vi "读取数据库.vi"(7 "condition":string, 8 "error in (no error)":errorcluster caption="错误输入（无错误）", 9 "database":string="database1.mdb", 10 "显示项":string[](array[string]), 11 "组合框":string(combo)) -> (0 "error out":errorcluster caption="错误输出", 1 "columns":string[](array[string]), 2 "data":variant[][](array[variant]), 3 "表格":string[][](table))   [LabVIEW 2016, in "数据查询.lvlib"]
uses:
  <vilib>/Utility/sysdir.llb/System Directory Type.ctl
  <vilib>/addons/database/Connection.llb/DB Tools Open Connec (String).vi
  <vilib>/addons/database/_DB Variant To Data/Database Variant To Data.xnode
  <vilib>/addons/database/NI_Database_API.lvlib
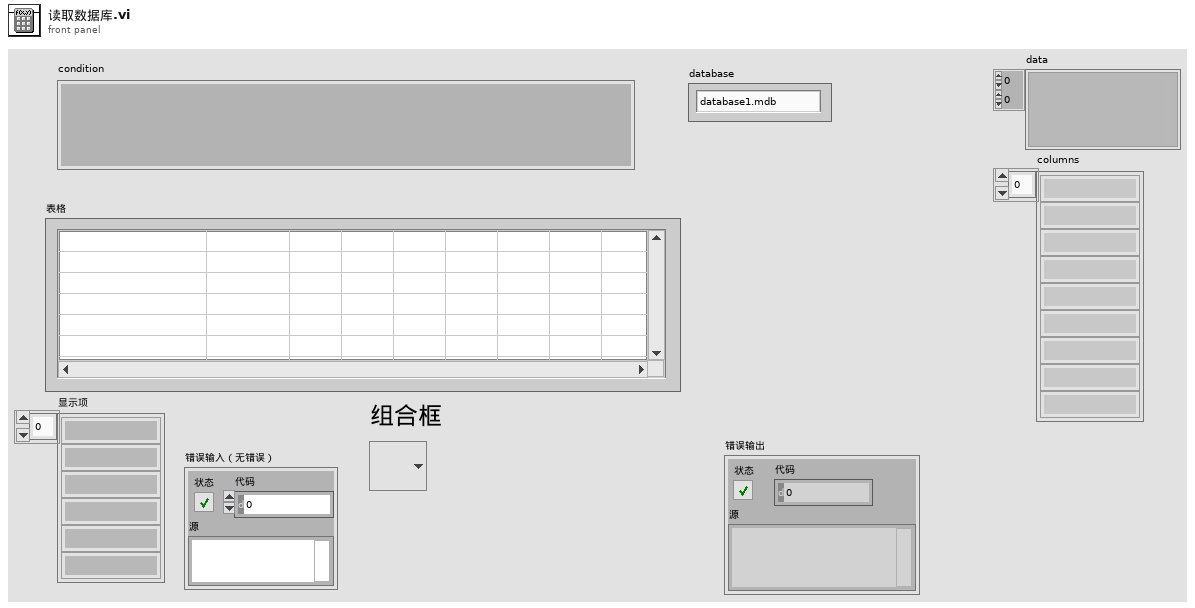
[diagram p1: front panel]
types:
  T1 = typedef "System Directory Type.ctl" = i32
  T2 = typedef "NI_Database_API.lvlib/Conn ObjectReference.ctl" = refnum<k1>
  T3 = typedef "NI_Database_API.lvlib/DB Tools DataTypes.ctl" = enum16{"String", "Long (I32)", "Single (SGL)", "Double (DBL)", "Date/Time", "Binary"}
  T4 = cluster{"name":string, "database data type":T3, "defined size":i32}[]
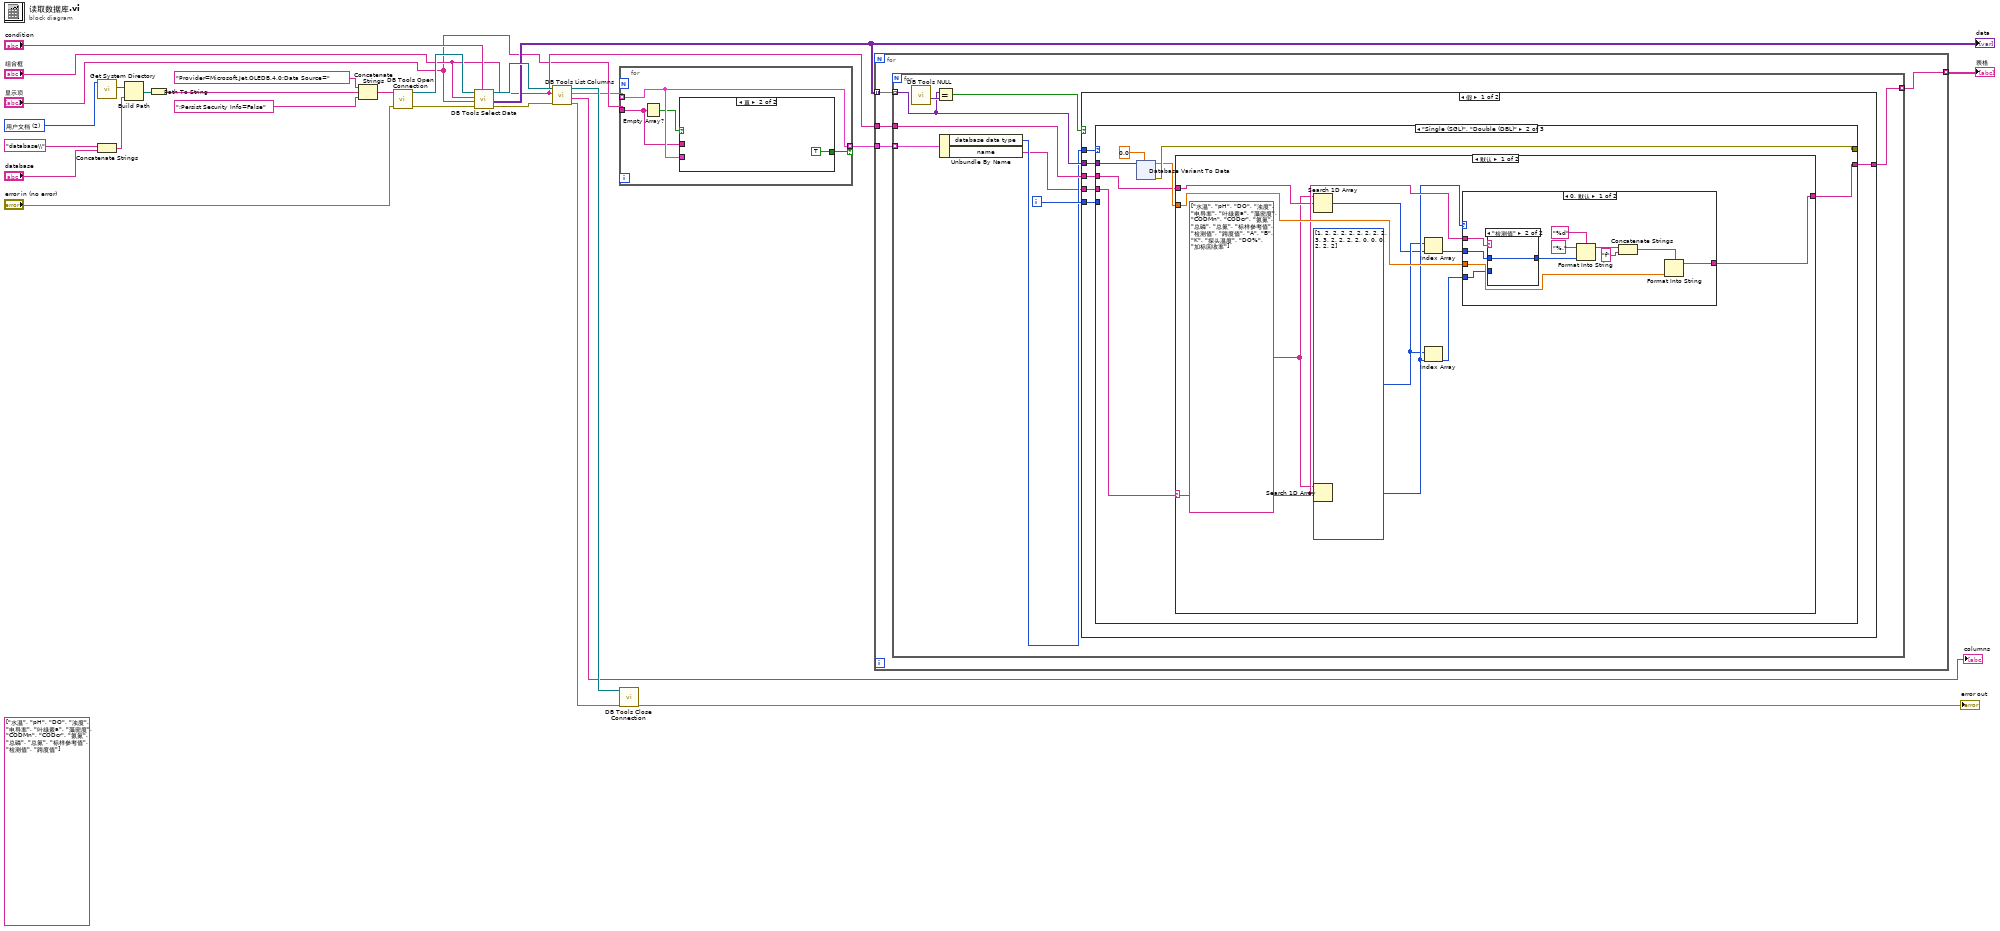
[diagram p0: block diagram]
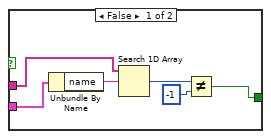
[diagram p2: hidden frame]
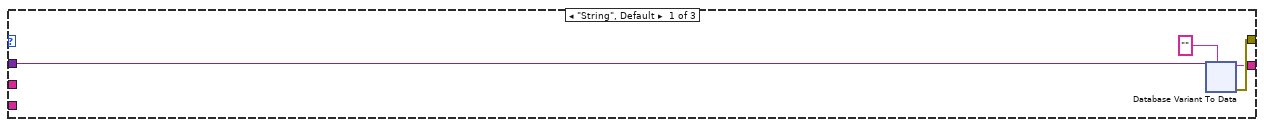
[diagram p3: hidden frame]
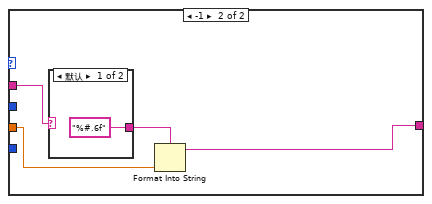
[diagram p5: hidden frame]
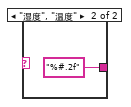
[diagram p6: hidden frame]
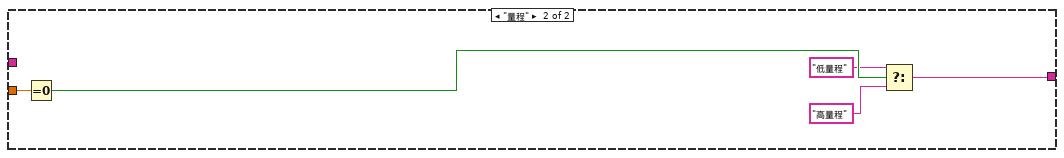
[diagram p7: hidden frame]
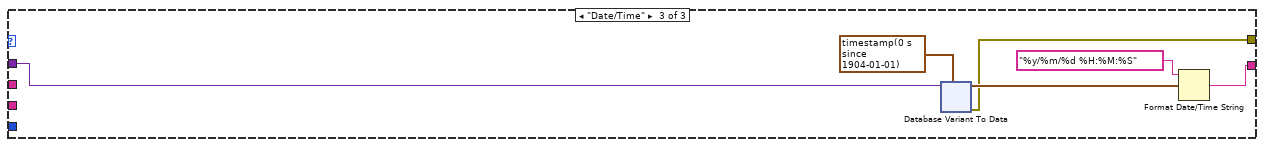
[diagram p8: hidden frame]
diagram:
  (unwired) string[] ["水温", "pH", "DO", "浊度", "电导率", "叶绿素a", "藻密度", "CODMn", "CODcr", "氨氮", "总磷", "总氮", "标样参考值", "检测值", "跨度值"]
  w13 = T1 2 items=["用户目录"=0, "用户桌面"=1, "用户文档"=2, "用户应用程序数据"=3, "用户设置"=4, "用户临时目录"=5, "公共文档"=6, "公共应用程序数据"=7, "公共设置"=8, "公共缓存"=13, "系统核心库"=9, "系统安装库"=10, "应用程序文件"=11, "启动盘根目录"=12] ("system directory type")
  n1 = call <vilib>:"Get System Directory.vi"("system directory type"=w13) -> ("system directory"=w12:path)  [unwired: 10 in]
  n2 = Concatenate Strings("database\\" ("名称或相对路径"), "database") -> (w9:string)
  n3 = Build Path(base path=w12, name or relative path=w9) -> (appended path=w14:path)
  n4 = Path To String(path=w14) -> (string=w15:string)
  n5 = Concatenate Strings("Provider=Microsoft.Jet.OLEDB.4.0;Data Source=", w15, ";Persist Security Info=False") -> (w11:string)
  n6 = call-poly <vilib>:"DB Tools Open Connection.vi"("error in (no error)"="error in (no error)", "connection information"=w11) -> ("error out"=w25:errorcluster, "connection reference"=w26:T2)  [unwired: 6 in]
  n7 = call <vilib>:"DB Tools Select Data.vi"("condition"="condition", "error in (no error)"=w25, "columns"="显示项", "table"="组合框", "connection reference"=w26) -> ("error out"=w24:errorcluster, "data"=w7:variant[][], "connection reference out"=w21:T2)  [unwired: 1 in]
  "data" <- w7
  n8 = call <vilib>:"DB Tools List Columns.vi"("error in (no error)"=w24, "table"="组合框", "connection reference"=w21) -> ("error out"=w18:errorcluster, "columns"=→"columns":string[], "column information"=w2:T4, "connection reference out"=w19:T2)  [unwired: 1 in]
  n9 = for {
    tunnel: w2 -> [w29] mode=indexing
    tunnel: "显示项" -> [w28]
    tunnel: [w29] -> w1 mode=indexing if=w30
    n10 = Empty Array?(array=w28) -> (empty?=w27:bool)
    n11 = case shown="真" w27 {
      tunnel: [w33 TRUE] -> w30
      tunnel: w29 -> [w32 _]
      tunnel: w28 -> [w31 _]
      frame False {
        n12 = Unbundle By Name(w32) -> ("name"=w34:string)
        n13 = Search 1D Array(1D array=w31, element=w34) -> (index of element=w36:i32)  [unwired: 1 in]
        n14 = Not Equal?(x=w36, y=-1) -> (x != y?=w33:bool)
      }
      frame True {
      }
    }
  }
  n15 = call <vilib>:"DB Tools Close Connection.vi"("error in (no error)"=w18, "connection reference"=w19) -> ("error out"=→"error out":errorcluster)  [unwired: 5 in]
  n16 = for {
    tunnel: w7 -> [w41] mode=indexing
    tunnel: w1 -> [w40]
    tunnel: [w39] -> w6 mode=indexing
    tunnel: "组合框" -> [w38]
    n17 = for {
      tunnel: w41 -> [w46] mode=indexing
      tunnel: w40 -> [w50] mode=indexing
      tunnel: [w48] -> w39 mode=indexing
      tunnel: w38 -> [w44]
      i -> [w49]
      n18 = call <vilib>:"DB Tools NULL.vi"() -> ("NULL"=w47:variant)  [unwired: 10 in, 1 out]
      n19 = Equal?(x=w46, y=w47) -> (x = y?=w45:bool)
      n20 = Unbundle By Name(w50) -> ("database data type"=w43:T3, "name"=w42:string)
      n21 = case shown="假" w45 {
        tunnel: w43 -> [w56 _]
        tunnel: w49 -> [w55 _]
        tunnel: [w54 _] -> w48
        tunnel: w42 -> [w53 _]
        tunnel: w46 -> [w52 _]
        tunnel: w44 -> [w51 _]
        frame False {
          n22 = case shown="\"Single (SGL)\", \"Double (DBL)\"" w56 {
            tunnel: w52 -> [w60 w97 w171]
            tunnel: [w57 w98 w167] -> w54
            tunnel: w55 -> [_ _ _]
            tunnel: [w58 w99 w166] -> _
            tunnel: w53 -> [_ w96 _]
            tunnel: w51 -> [_ w93 _]
            frame "String", Default {
              n23 = xnode "Database Variant To Data"("database variant"=w60, "type"="") -> ("data"=w57:string, "error out"=w58:errorcluster)  [unwired: 1 in]
            }
            frame "Single (SGL)", "Double (DBL)" {
              n24 = xnode "Database Variant To Data"("database variant"=w97, "type"=0.0) -> ("data"=w94:dbl, "error out"=w99:errorcluster)  [unwired: 1 in]
              n25 = case shown="默认" w96 {
                selector: w96 -> [w107 _]
                tunnel: w94 -> [w109 w133]
                tunnel: [w108 w129] -> w98
                tunnel: w93 -> [w105 _]
                frame Default {
                  w100 = string[] ["水温", "pH", "DO", "浊度", "电导率", "叶绿素a", "藻密度", "CODMn", "CODcr", "氨氮", "总磷", "总氮", "标样参考值", "检测值", "跨度值", "A", "B", "K", "探头温度", "DO%", "加标回收率"]
                  w104 = i32[] [1, 2, 2, 2, 2, 2, 2, 2, 2, 3, 3, 2, 2, 2, 2, 0, 0, 0, 2, 2, 2]
                  n26 = Search 1D Array(1D array=w100, element=w105) -> (index of element=w103:i32)  [unwired: 1 in]
                  n27 = Search 1D Array(1D array=w100, element=w107) -> (index of element=w106:i32)  [unwired: 1 in]
                  n28 = Index Array(array=w104, index=w103) -> (element=w102:i32)
                  n29 = Index Array(array=w104, index=w106) -> (element=w101:i32)
                  n30 = case shown="0, 默认" w106 {
                    tunnel: w109 -> [w114 w126]
                    tunnel: [w112 w125] -> w108
                    tunnel: w107 -> [w113 w123]
                    tunnel: w102 -> [w111 _]
                    tunnel: w101 -> [w110 _]
                    frame 0, Default {
                      n31 = case shown="\"检测值\"" w113 {
                        tunnel: [w121 w122] -> w120
                        tunnel: w111 -> [_ w122]
                        tunnel: w110 -> [w121 _]
                        frame Default {
                        }
                        frame "检测值" {
                        }
                      }
                      n32 = Format Into String(format string="%d" ("格式字符串"), initial string="%." ("初始字符串"), w120) -> (resulting string=w118:string)  [unwired: 1 in, 1 out]
                      n33 = Concatenate Strings(w118, "f" ("格式字符串")) -> (w116:string)
                      n34 = Format Into String(format string=w116, w114) -> (resulting string=w112:string)  [unwired: 2 in, 1 out]
                    }
                    frame -1 {
                      n35 = case shown="默认" w123 {
                        tunnel: ["%#.6f" ("格式字符串") "%#.2f" ("格式字符串")] -> w124
                        frame Default {
                        }
                        frame "湿度", "温度" {
                        }
                      }
                      n36 = Format Into String(format string=w124, w126) -> (resulting string=w125:string)  [unwired: 2 in, 1 out]
                    }
                  }
                }
                frame "量程" {
                  n37 = Equal To 0?(x=w133) -> (x = 0?=w132:bool)
                  n38 = Select(t="低量程" ("格式字符串"), s=w132, f="高量程" ("格式字符串")) -> (s? t:f=w129:string)
                }
              }
            }
            frame "Date/Time" {
              n39 = xnode "Database Variant To Data"("database variant"=w171, "type"=timestamp(0 s since 1904-01-01) ("当前时间")) -> ("data"=w170:timestamp, "error out"=w166:errorcluster)  [unwired: 1 in]
              n40 = Format Date/Time String(time format string (%c)="%y/%m/%d %H:%M:%S" ("时间格式字符串(%c)"), seconds (now)=w170) -> (date/time string=w167:string)  [unwired: 1 in]
            }
          }
        }
        frame True {
        }
      }
    }
  }
  "表格" <- w6
